vi "CreateAnchor.vi"(1 "Anchor Y":dbl, 2 "Anchor X":dbl, 3 "Anchor ID":dbl) -> (0 "Anchor Out":refnum<class "Anchor.lvclass">)   [LabVIEW 2014, in "Anchor.lvclass"]
uses:
  Anchor.lvclass
  Anchor.lvclass/Anchor.ctl
panel:
  out "error out":errorcluster
  in  "error in (no error)":errorcluster
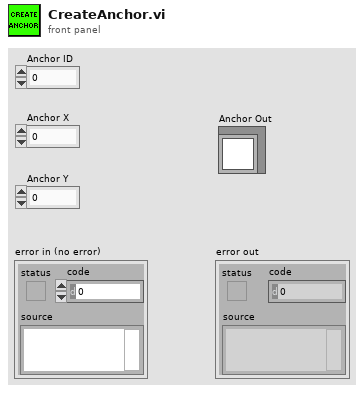
[diagram p1: front panel]
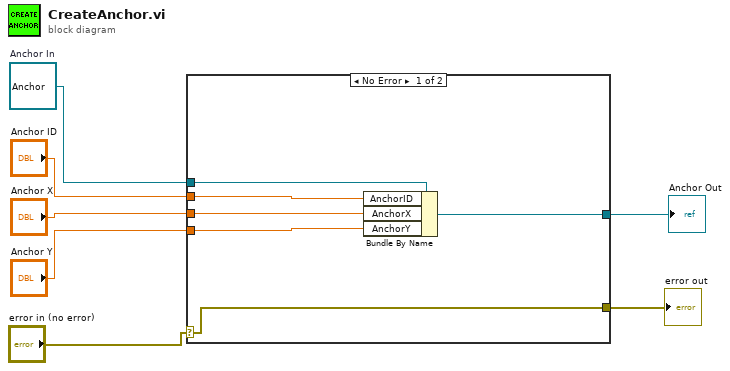
[diagram p0: block diagram]
diagram:
  w3 = refnum<class "Anchor.lvclass"> refnum  # Anchor In
  n1 = case shown="No Error" "error in (no error)" {
    selector: "error in (no error)" -> [w9 w14]
    tunnel: "Anchor ID" -> [w13 _]
    tunnel: "Anchor X" -> [w12 _]
    tunnel: "Anchor Y" -> [w11 _]
    tunnel: w3 -> [w10 w15]
    tunnel: [w9 w14] -> w2
    tunnel: [w8 w15] -> w1
    frame No Error {
      n2 = Bundle By Name(cluster=w10, "AnchorID"=w13, "AnchorX"=w12, "AnchorY"=w11) -> (w8:refnum<class "Anchor.lvclass">)
    }
    frame Error {
    }
  }
  "error out" <- w2
  "Anchor Out" <- w1
